vi "Do.vi"(8 "error in (no error)":errorcluster, 10 "Actor in":refnum<class "Actor.lvclass">, 11 "Function Done":refnum<class "Function Done.lvclass">) -> (0 "error out":errorcluster, 2 "Actor out":refnum<class "Actor.lvclass">)   [LabVIEW 2016, in "Controller Actor.lvlib" / "Function Done.lvclass"]
uses:
  <userlib>/Common Components/Controller/Messages/Function Done Message/Function Done.lvclass
  <vilib>/ActorFramework/Actor/Actor.lvclass
  <userlib>/Common Components/Controller/Controller.lvclass
  C:/Program Files (x86)/National Instruments/LabVIEW 2016/vi.lib/ActorFramework/Actor/Actor.lvclass
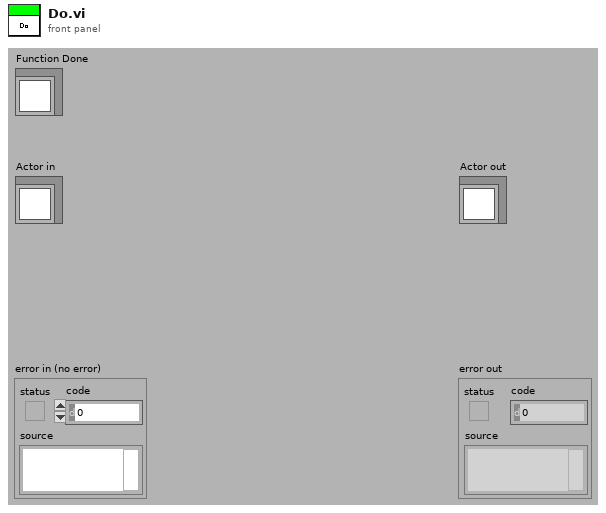
[diagram p1: front panel]
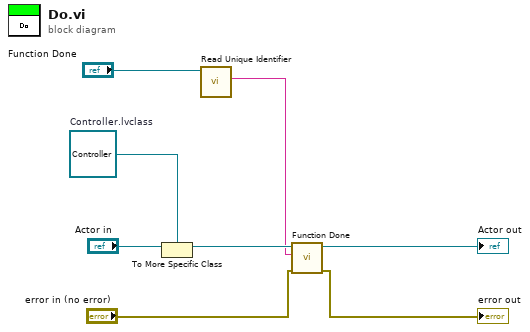
[diagram p0: block diagram]
diagram:
  w3 = refnum<class "Controller.lvclass"> refnum  # Controller.lvclass
  n1 = To More Specific Class(target class=w3, reference="Actor in") -> (specific class reference=w7:refnum<class "Controller.lvclass">)  [unwired: 1 in, 1 out]
  n2 = call <userlib>:"Read Unique Identifier.vi"("Function Done in"="Function Done") -> ("Unique Identifier"=w5:string)  [unwired: 8 in, 2 out]
  n3 = call-dynamic "Function Done.vi"("error in (no error)"="error in (no error)", "GUID"=w5, "Controller in"=w7) -> ("error out"=→"error out":errorcluster, "Controller out"=→"Actor out":refnum<class "Controller.lvclass">)  [unwired: 7 in]
